vi "SetParam.vi"(8 "error in (no error)":errorcluster caption="entrée d'erreur (pas d'erreur)", 10 "label_ranking_loss":cluster{"sample_weight":dbl[]}, 11 "Label_Ranking_Loss.lvclass":refnum<class "Label_Ranking_Loss.lvclass">) -> (0 "error out":errorcluster caption="sortie d'erreur", 3 "Label_Ranking_Loss.lvclass":refnum<class "Label_Ranking_Loss.lvclass">)   [LabVIEW 2020, in "Label_Ranking_Loss.lvclass"]
doc: "Set Parameters"
uses:
  Label_Ranking_Loss.lvclass
  Label_Ranking_Loss.lvclass/Label_Ranking_Loss.ctl
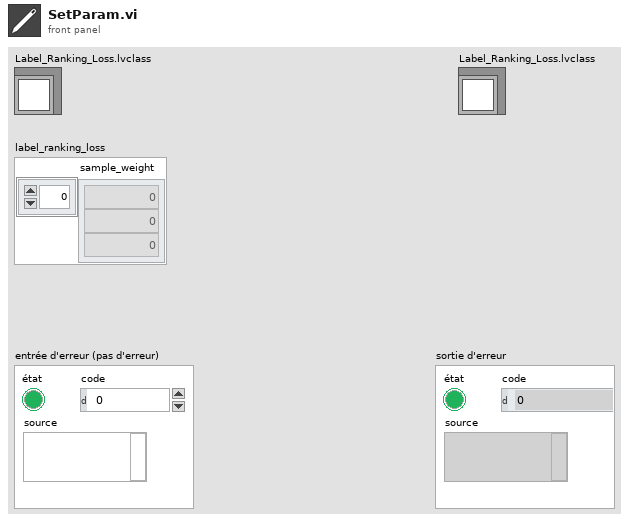
[diagram p1: front panel]
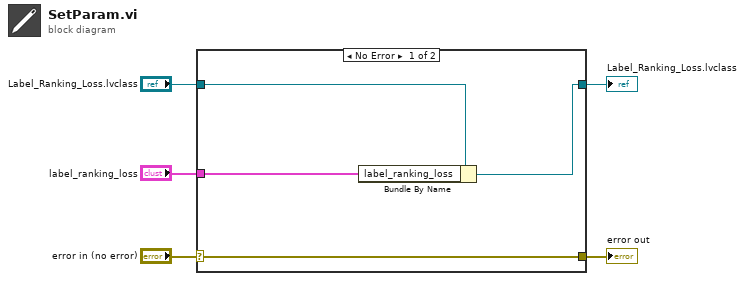
[diagram p0: block diagram]
diagram:
  n1 = case shown="No Error" "error in (no error)" {
    selector: "error in (no error)" -> [w9 w10]
    tunnel: [w9 w10] -> w4
    tunnel: [w7 w11] -> w2
    tunnel: "Label_Ranking_Loss.lvclass" -> [w8 w11]
    tunnel: "label_ranking_loss" -> [w6 _]
    frame No Error {
      n2 = Bundle By Name(cluster=w8, "label_ranking_loss"=w6) -> (w7:refnum<class "Label_Ranking_Loss.lvclass">)
    }
    frame Error {
    }
  }
  "error out" <- w4
  "Label_Ranking_Loss.lvclass" <- w2
